vi "New Test Case.vi"() -> ()   [LabVIEW 2011]
uses:
  Libraries/VITesterUtilities.lvlib
panel:
  out "error out":errorcluster
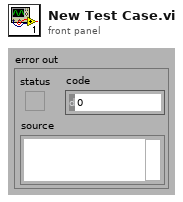
[diagram p1: front panel]
types:
  T1 = typedef "Menu Launch Info - Cluster__jki_lib_application_control -- VI Tester.ctl" = cluster{"Application":refnum<vi>, "Selected Project Items":T2[]}
  T2 = typedef "Project Item Info - Cluster__jki_lib_application_control -- VI Tester.ctl" = cluster{"Type":string, "Name":string, "Path":path}
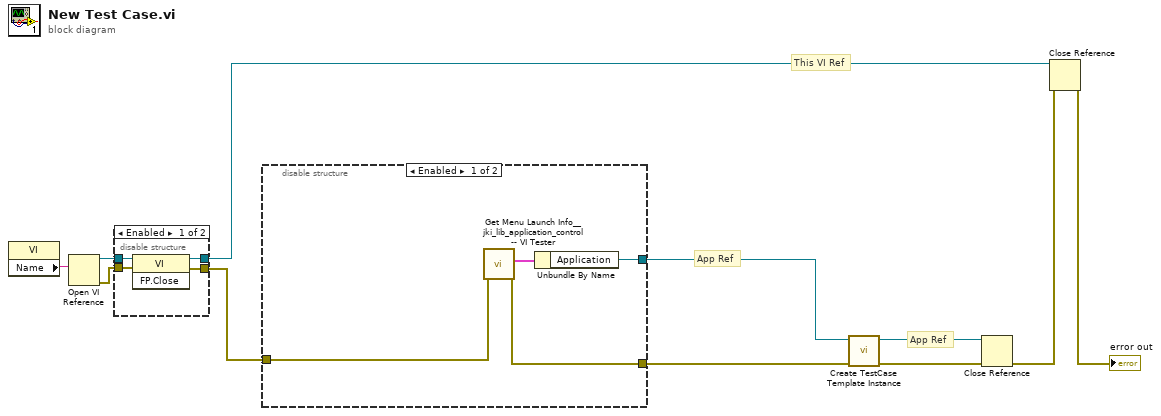
[diagram p0: block diagram]
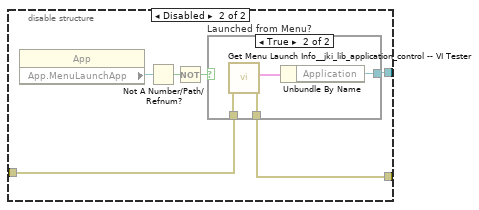
[diagram p2: hidden frame]
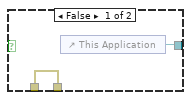
[diagram p3: hidden frame]
diagram:
  # "App Ref"
  # "App Ref"
  # "This VI Ref"
  n1 = property class="VI"() -> ("Name"=w11:string)  [unwired: 2 in, 2 out]
  n2 = Open VI Reference(vi path=w11) -> (vi reference=w10:refnum<vi>, error out=w8:errorcluster)  [unwired: 5 in]
  n3 = disable-structure shown="Enabled" {
    disable-tunnel: [w15 w16] -> w3
    disable-tunnel: w10 -> [w14 w17]
    disable-tunnel: [w13 w17] -> w9
    disable-tunnel: w8 -> [w12 w16]
    frame Enabled {
      n4 = invoke class="VI" method="FP.Close"(reference=w14, error in=w12) -> (reference out=w13:refnum<vi>, error out=w15:errorcluster)  [unwired: 1 in, 1 out]
    }
    frame Disabled {
    }
  }
  n5 = disable-structure shown="Enabled" {
    disable-tunnel: w3 -> [w21 w24]
    disable-tunnel: [w20 w23] -> w1
    disable-tunnel: [w19 w22] -> w2
    frame Enabled {
      n6 = call "Get Menu Launch Info__jki_lib_application_control -- VI Tester.vi"("error in (no error)"=w21) -> ("error out"=w20:errorcluster, "Menu Launch info"=w18:T1)  [unwired: 9 in]
      n7 = Unbundle By Name(w18) -> ("Application"=w19:refnum<vi>)
    }
    frame Disabled {
      n8 = property class="App"() -> ("App.MenuLaunchApp"=w27:refnum<vi>)  [unwired: 2 in, 2 out]
      n9 = Not A Number/Path/Refnum?(number/path/refnum=w27) -> (NaN/Path/Refnum?=w26:bool)
      n10 = Not(x=w26) -> (.not. x?=w25:bool)
      n11 = case "Launched from Menu?" shown="True" w25 {
        tunnel: [w29 w32] -> w22
        tunnel: [w28 w31] -> w23
        tunnel: w24 -> [w28 w30]
        frame False {
          n12 = control-ref of="This Application"() -> (w29:refnum<vi>)
        }
        frame True {
          n13 = call "Get Menu Launch Info__jki_lib_application_control -- VI Tester.vi"("error in (no error)"=w30) -> ("error out"=w31:errorcluster, "Menu Launch info"=w33:T1)  [unwired: 9 in]
          n14 = Unbundle By Name(w33) -> ("Application"=w32:refnum<vi>)
        }
      }
    }
  }
  n15 = call "Create TestCase Template Instance.vi"("error in"=w1, "Application Ref (This Application)"=w2) -> ("error out"=w5:errorcluster, "Application Ref"=w4:refnum<vi>)  [unwired: 8 in]
  n16 = Close Reference(reference=w4, error in (no error)=w5) -> (error out=w7:errorcluster)
  n17 = Close Reference(reference=w9, error in (no error)=w7) -> (error out=→"error out":errorcluster)
